vi "MicroDAQ_UDP.vi"() -> ()   [LabVIEW 2021]
uses:
  <vilib>/Analysis/baseanly.llb/Mean (DBL).vi
  <vilib>/DAQmx/create/channels.llb/DAQmx Create Channel (CO-Pulse Generation-Frequency).vi
  <vilib>/DAQmx/configure/timing.llb/DAQmx Timing (Implicit).vi
  <vilib>/Analysis/NI_AALBase.lvlib
  <resource>/objmgr/daqmx.rc
panel:
  in  "Local IP":string="192.168.1.183"
  out "Command Packet Byte String":string
  in  "CO.Pulse.Term":tag
  out "error out":errorcluster
  out "Waveform Chart":dbl(graph)
  out "Loop index":i32
  in  "frequency":dbl=250.0
  out "Local port":u16
  out "Remote port":u16
  out "Remote IP":string
  in  "counter":tag="PXI1Slot2/ctr0"
  in  "stop":bool
  out "data out":string
  in  "Remote IP":string="192.168.1.190"
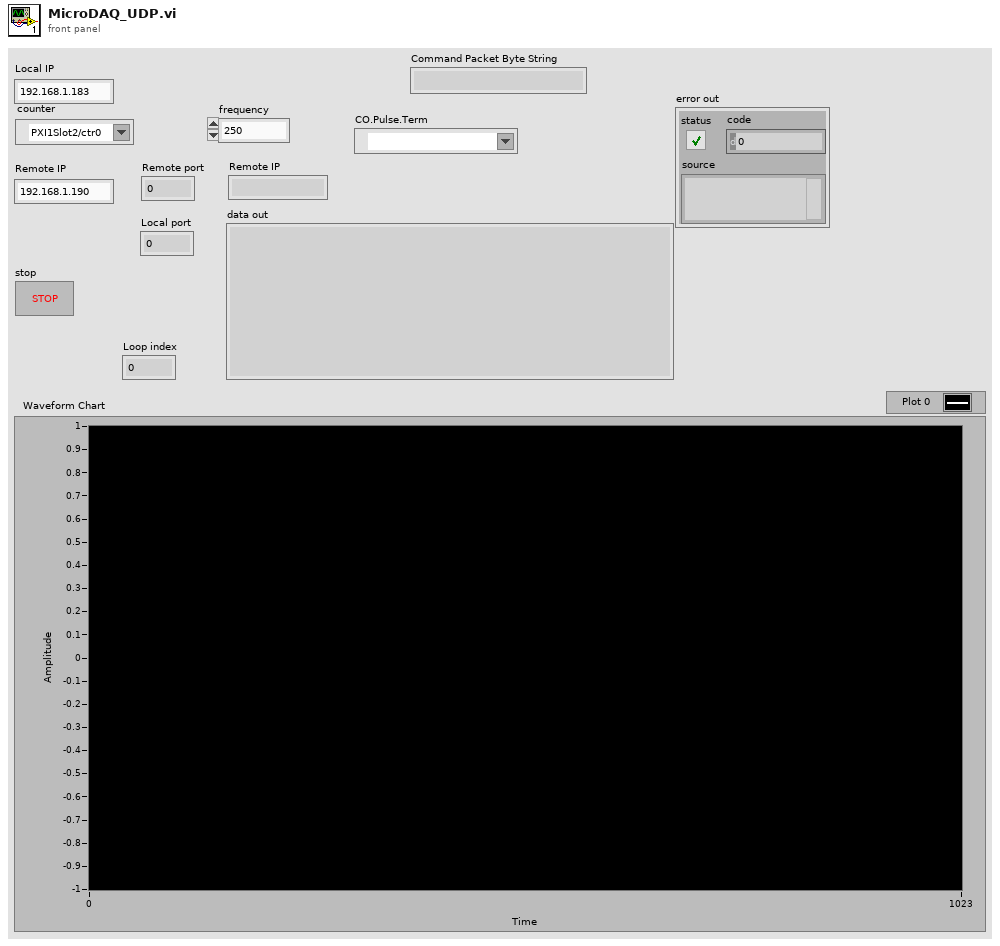
[diagram p1: front panel]
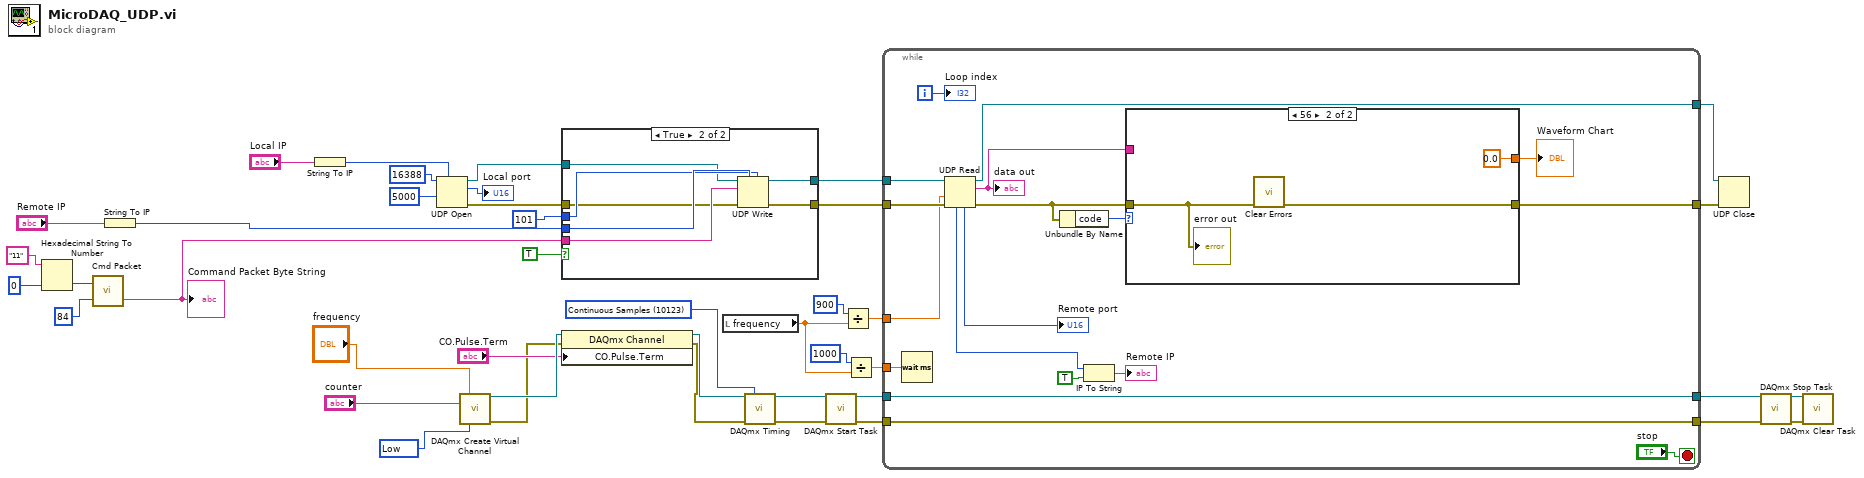
[diagram p0: block diagram]
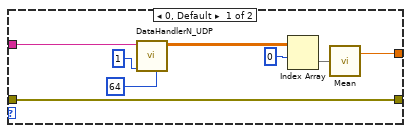
[diagram p3: hidden frame]
diagram:
  w38 = 10123 items=["Finite Samples"=10178, "Continuous Samples"=10123, "Hardware Timed Single Point"=12522] ("sample mode")
  w39 = 10214 items=["High"=10192, "Low"=10214] ("idle state")
  n1 = Hexadecimal String To Number(string="11" ("Hardware Trigger"), default (0uL)=i8 0 ("default (0 U32)")) -> (number=w27:i8)  [unwired: 1 in, 1 out]
  n2 = call "Cmd Packet.vi"("Command Byte"=84 ("data in"), "Parameter Byte"=w27) -> ("Command Packet Byte String"=w26:string)  [unwired: 1 out]
  "Command Packet Byte String" <- w26
  n3 = String To IP(1:"Remote IP") -> (0:w24:u32)
  n4 = String To IP(1:"Local IP") -> (0:w4:u32)
  n5 = UDP Open(7:w4, 9:5000 ("timeout ms (25000)"), 11:u16 16388 ("port")) -> (port=w22:refnum<k16>, 0:w21:errorcluster, 2:→"Local port":u16)  [unwired: 2 in]
  n6 = call-poly <vilib>:"DAQmx Create Virtual Channel.vi"("frequency"="frequency", "counter"="counter", "idle state"=w39) -> ("task out"=w9:refnum<k21>, "error out"=w2:errorcluster)  [unwired: 11 in]
  n7 = case shown="True" TRUE {
    tunnel: w26 -> [_ w51]
    tunnel: w24 -> [_ w50]
    tunnel: u16 101 ("port or service name") -> [_ w49]
    tunnel: w22 -> [w44 w48]
    tunnel: w21 -> [w43 w47]
    tunnel: [w43 w46] -> w20
    tunnel: [w44 w45] -> w19
    frame False {
    }
    frame True {
      n8 = UDP Write(address=w50, port or service name=w49, connection ID=w48, data in=w51, 8:w47) -> (error out=w46:errorcluster, 3:w45:refnum<k16>)  [unwired: 1 in]
    }
  }
  n9 = property class="DAQmx Channel"(reference=w9, error in=w2, "CO.Pulse.Term"="CO.Pulse.Term") -> (reference out=w8:refnum<k21>, error out=w1:errorcluster)
  n10 = local read "frequency"() -> (w10:dbl)
  n11 = call-poly <vilib>:"DAQmx Timing.vi"("task/channels in"=w8, "sample mode"=w38, "error in"=w1) -> ("task out"=w33:refnum<k21>, "error out"=w32:errorcluster)  [unwired: 11 in]
  n12 = call <vilib>:"DAQmx Start Task.vi"("task/channels in"=w33, "error in"=w32) -> ("task out"=w15:refnum<k21>, "error out"=w17:errorcluster)  [unwired: 12 in]
  n13 = Divide(x=900 ("timeout ms (25000)"), y=w10) -> (x/y=w12:dbl)
  n14 = Divide(x=1000 ("timeout ms (25000)"), y=w10) -> (x/y=w3:dbl)
  n15 = while {
    tunnel: w20 -> [w69]
    tunnel: w19 -> [w68]
    tunnel: [w62] -> w41
    tunnel: [w67] -> w40
    tunnel: [w60] -> w16
    tunnel: w17 -> [w60]
    tunnel: w15 -> [w59]
    tunnel: [w59] -> w14
    tunnel: w12 -> [w52]
    tunnel: w3 -> [w53]
    i -> [w61]
    stop <- "stop" stop-if-true
    n16 = Wait (ms)(milliseconds to wait=w53) -> ()  [unwired: 1 out]
    n17 = UDP Read(connection ID=w68, timeout ms (25000)=w52, 8:w69) -> (data out=w58:string, error out=w56:errorcluster, 3:w67:refnum<k16>, 4:→"Remote port":u16, 6:w66:u32)  [unwired: 1 in]
    "data out" <- w58
    n18 = Unbundle By Name(w56) -> ("code"=w55:i32)
    n19 = IP To String(1:TRUE ("dot notation? (F)"), 2:w66) -> (0:→"Remote IP":string)
    n20 = case shown="56" w55 {
      tunnel: w56 -> [w70 w80]
      tunnel: [w70 w79] -> w62
      tunnel: w58 -> [w75 _]
      tunnel: [w74 0.0] -> w57
      frame 0, Default {
        n21 = call "DataHandlerN_UDP.vi"("Data Cycles Per Buffer"=1, "data out"=w75, "Nchan"=64) -> ("Data"=w73:sgl[][])  [unwired: 2 in, 4 out]
        n22 = Index Array(array=w73, index (row)=0 ("Data Cycles Per Buffer")) -> (element=w71:sgl[])  [unwired: 1 in]
        n23 = call-poly <vilib>:"Mean.vi"("X"=w71) -> ("mean"=w74:dbl)  [unwired: 1 out]
      }
      frame 56 {
        n24 = call <vilib>:"Clear Errors.vi"("error in (no error)"=w80) -> ("error out"=w79:errorcluster)  [unwired: 5 in, 1 out]
        "error out" <- w80
      }
    }
    "Waveform Chart" <- w57
    "Loop index" <- w61
  }
  n25 = UDP Close(connection ID=w40, 8:w41) -> ()  [unwired: 2 out]
  n26 = call <vilib>:"DAQmx Stop Task.vi"("task/channels in"=w14, "error in"=w16) -> ("task out"=w36:refnum<k21>, "error out"=w37:errorcluster)  [unwired: 12 in]
  n27 = call <vilib>:"DAQmx Clear Task.vi"("task in"=w36, "error in"=w37) -> ()  [unwired: 13 in, 1 out]
